vi "joystick new.vi"() -> ()   [LabVIEW 2020]
uses:
  Communication_class/Paths/Convert AI Robot to Robot Command Folder/grSim/grSim Robot Command.ctl
  <vilib>/Analysis/baseanly.llb/Unit Vector (DBL).vi
  <vilib>/Instr/_visa.llb/VISA Configure Serial Port (Instr).vi
  <vilib>/Analysis/NI_AALBase.lvlib
panel:
  in  "v_ang_max":dbl=4.0 format="%#_13g"
  in  "v_max":dbl=1.0
  in  "id":u32
  out "Visa return count":u32
  out "String":string
  out "return count":u32
  in  "stop":bool
  out "string":string
  out "error out":errorcluster
  in  "termination char\n(0xA = '\\n' = LF)":u8=10 format="%.0x"
  in  "VISA resource name":refnum<visa-resource-name>
  in  "Serial Settings":T1={"baud rate"=9600, "data bits"=8, "parity"=enum."None", "stop bits"=10, "flow control"=0} {"flow control" items=["None"=0, "XON/XOFF"=1, "RTS/CTS"=2, "DTR/DSR"=4]; "stop bits" items=["1.0"=10, "1.5"=15, "2.0"=20]; "data bits" min=5 max=8 step=1; "baud rate" items=["75"=75, "110"=110, "134"=134, "150"=150, "300"=300, "600"=600, "1200"=1200, "1800"=1800, "2400"=2400, "4800"=4800, "7200"=7200, "9600"=9600, "14400"=14400, "19200"=19200, "28800"=28800, "38400"=38400, "56000"=56000, "57600"=57600, "115200"=115200, "128000"=128000, "230400"=230400]}
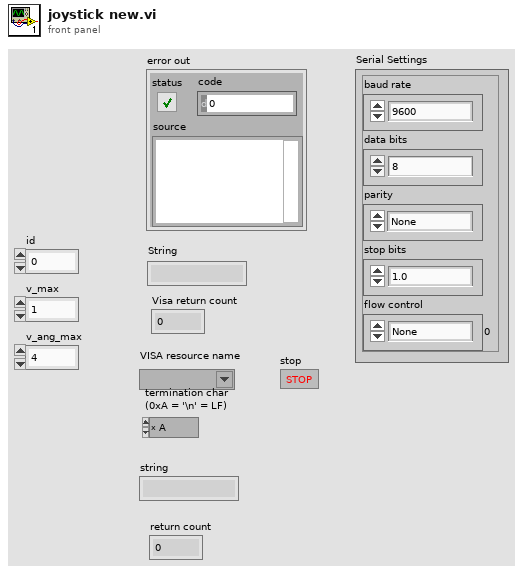
[diagram p1: front panel]
types:
  T1 = cluster{"baud rate":u32, "data bits":u16, "parity":enum16{"None", "Odd", "Even", "Mark", "Space"}, "stop bits":u16, "flow control":u16}
  T2 = typedef "grSim Robot Command.ctl" = cluster{"id":u32, "kickspeedx":sgl, "kickspeedz":sgl, "veltangent":sgl, "velnormal":sgl, "velangular":sgl, "spinner":bool, "wheelspeed":bool, "wheel1":sgl, "wheel2":sgl, "wheel3":sgl, "wheel4":sgl, "kickangle":sgl, "spinner_rpm":sgl}
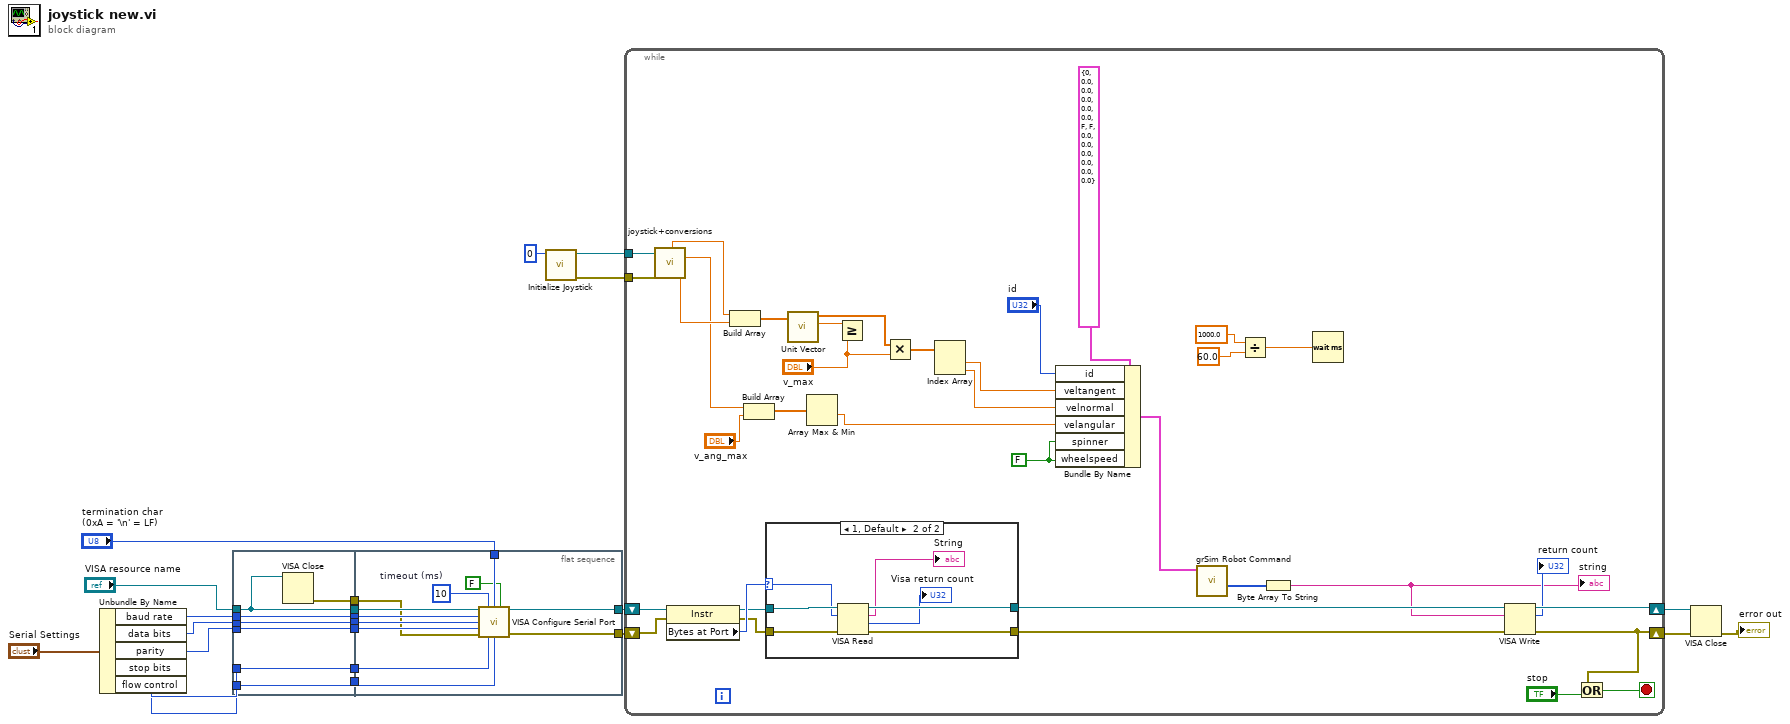
[diagram p0: block diagram]
diagram:
  n1 = Unbundle By Name("Serial Settings") -> ("baud rate"=w22:u32, "data bits"=w21:u16, "parity"=w20:enum16{"None", "Odd", "Even", "Mark", "Space"}, "stop bits"=w19:u16, "flow control"=w18:u16)
  n2 = flat-sequence {
    tunnel: "VISA resource name" -> [w25]
    tunnel: w18 -> [w26]
    tunnel: w19 -> [w27]
    tunnel: w20 -> [w28]
    tunnel: w21 -> [w29]
    tunnel: w22 -> [w30]
    tunnel: [w30] -> w10
    tunnel: [w29] -> w9
    tunnel: [w28] -> w8
    tunnel: [w27] -> w7
    tunnel: [w26] -> w6
    tunnel: [w25] -> w5
    tunnel: [w24] -> w4
    tunnel: "termination char\n(0xA = '\\n' = LF)" -> [w36]
    tunnel: [w34] -> w15
    tunnel: [w33] -> w13
    tunnel: w10 -> [w42]
    tunnel: w9 -> [w41]
    tunnel: w8 -> [w40]
    tunnel: w7 -> [w39]
    tunnel: w6 -> [w38]
    tunnel: w5 -> [w37]
    tunnel: w4 -> [w31]
    frame #0 {
      n3 = VISA Close(VISA resource name=w25) -> (error out=w24:errorcluster)  [unwired: 1 in]
    }
    frame #1 {
      w32 = u32 10  # timeout (ms)
      n4 = call-poly "VISA Configure Serial Port"("VISA resource name"=w37, "timeout (10sec)"=w32, "termination char\n(0xA = '\\n' = LF)"=w36, "Enable Termination\nChar (T)"=FALSE ("Enable Termination\nChar (T)"), "baud rate (9600)"=w42, "data bits (8)"=w41, "parity (0:none)"=w40, "error in (no error)"=w31, "stop bits (10: 1 bit)"=w39, "flow control (0:none)"=w38) -> ("VISA resource name out"=w34:refnum<visa-resource-name>, "error out"=w33:errorcluster)  [unwired: 4 in]
    }
  }
  n5 = call <vilib>:"Initialize Joystick.vi"("device index"=0) -> ("error out"=w1:errorcluster, "device ID"=w2:refnum<k1>)  [unwired: 9 in]
  n6 = while {
    shift-right: [w78] -> w14
    shift-left: w15 -> [w72]
    shift-right: [w75] -> w12
    shift-left: w13 -> [w71]
    tunnel: w2 -> [w61]
    tunnel: w1 -> [w60]
    stop <- w76 stop-if-true
    w62 = FALSE
    n7 = call "joystick+conversions.vi"("Refnum in"=w61, "error in (no error)"=w60) -> ("v_radial"=w55:dbl, "v_normal"=w54:dbl, "R*w"=w46:dbl)  [unwired: 9 in, 14 out]
    n8 = property class="Instr"(reference=w72, error in=w71) -> (reference out=w68:refnum<visa-resource-name>, error out=w69:errorcluster, "Bytes at Port"=w70:u32)
    n9 = Build Array(w55, w54) -> (w53:dbl[])
    n10 = Build Array(w46, "v_ang_max") -> (w44:dbl[])
    n11 = case shown="1, Default" w70 {
      selector: w70 -> [_ w81]
      tunnel: w69 -> [w79 w87]
      tunnel: [w79 w86] -> w74
      tunnel: w68 -> [w80 w85]
      tunnel: [w80 w84] -> w73
      frame 0 {
      }
      frame 1, Default {
        n12 = VISA Read(VISA resource name=w85, byte count=w81, error in (no error)=w87) -> (VISA resource name out=w84:refnum<visa-resource-name>, read buffer=→"String":string, return count=→"Visa return count":u32, error out=w86:errorcluster)
      }
    }
    n13 = call-poly <vilib>:"Unit Vector.vi"("Input Vector"=w53) -> ("norm"=w52:dbl, "Unit Vector"=w51:dbl[])  [unwired: 8 in, 1 out]
    n14 = Array Max & Min(array=w44) -> (min value=w43:dbl)  [unwired: 3 out]
    n15 = Greater Or Equal?(x=w52, y="v_max") -> ()  [unwired: 1 out]
    n16 = Multiply(x=w51, y="v_max") -> (x*y=w49:dbl[])
    n17 = Index Array(array=w49) -> (element #1=w48:dbl, element #2=w47:dbl)  [unwired: 2 in]
    n18 = Bundle By Name(cluster=T2 {"id"=0, "kickspeedx"=0.0, "kickspeedz"=0.0, "veltangent"=0.0, "velnormal"=0.0, "velangular"=0.0, "spinner"=FALSE, "wheelspeed"=FALSE, "wheel1"=0.0, "wheel2"=0.0, "wheel3"=0.0, "wheel4"=0.0, "kickangle"=0.0, "spinner_rpm"=0.0} ("Robots"), "id"="id", "veltangent"=w48, "velnormal"=w47, "velangular"=w43, "spinner"=w62, "wheelspeed"=w62) -> (w59:T2)
    n19 = call "grSim Robot Command.vi"("Robots"=w59) -> ("Array"=w65:u8[])  [unwired: 10 in]
    n20 = Divide(x=1000.0, y=60.0) -> (x/y=w57:dbl)
    n21 = Byte Array To String(unsigned byte array=w65) -> (string=w66:string)
    "string" <- w66
    n22 = Wait (ms)(milliseconds to wait=w57) -> ()  [unwired: 1 out]
    n23 = VISA Write(VISA resource name=w73, write buffer=w66, error in (no error)=w74) -> (VISA resource name out=w78:refnum<visa-resource-name>, return count=→"return count":u32, error out=w75:errorcluster)
    n24 = Or(x=w75, y="stop") -> (x .or. y?=w76:bool)
  }
  n25 = VISA Close(VISA resource name=w14, error in (no error)=w12) -> (error out=→"error out":errorcluster)
